vi "Read Image.vi"(0 "image in":refnum<class "MSC Image.lvclass">, 1 "image path":path, 5 "error in (no error)":errorcluster, 8 "read image properties":bool, 10 "image properties path":path) -> (14 "image out":refnum<class "MSC Image.lvclass">, 19 "error out":errorcluster)   [LabVIEW 2014, in "MSC Image.lvclass"]
doc: "Reads an image from the HD. If \"read image properties\" is set to TRUE, a previously created property file (.ini) is read and applied to the image.\n\nSupported formats:\nWindows bitmaps, JPEG, JPEG 2000, Portable Network Graphics, Portable image format, Sun rasters, TIFF"
uses:
  MSC Image.lvclass
  MSC Image.lvclass/MSC Image.ctl
  controls/INI Image Properties.vi
  controls/Size.ctl
  controls/Image Type.ctl
  <userlib>/_OpenG.lib/file/file.llb/Strip Path Extension - Path__ogtk.vi
  Dependencies/x86/MSC I Process32.dll
  <vilib>/Utility/config.llb/NI_LVConfig.lvlib
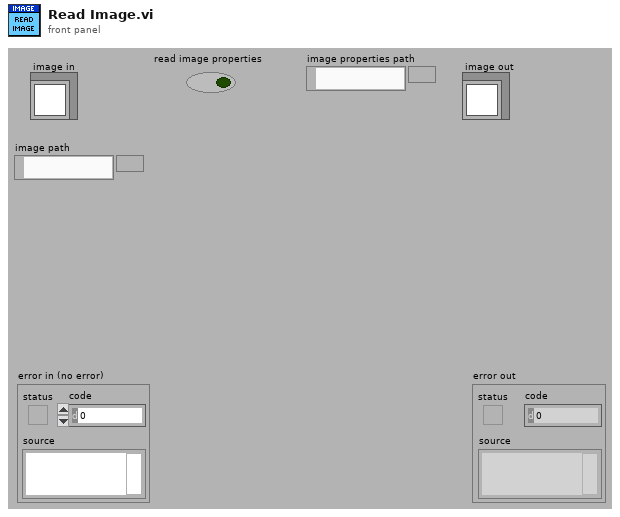
[diagram p1: front panel]
types:
  T1 = typedef "Image.ctl" = cluster{"Pointer":u64, "Size":T2, "Image Type":T3, "Time Stamp":timestamp, "Variant":variant}
  T2 = typedef "Size.ctl" = cluster{"Cols":i32, "Rows":i32}
  T3 = typedef "Image Type.ctl" = i32
  T4 = typedef "MSC Image.lvclass/INI Image Properties.vi" = cluster{"Size":T5, "Image Type":T6, "Timestamp":string, "Variant":variant}
  T5 = typedef "MSC Image.lvclass/Size.ctl" = cluster{"Cols":i32, "Rows":i32}
  T6 = typedef "MSC Image.lvclass/Image Type.ctl" = i32
  T7 = typedef "NI_LVConfig.lvlib/Config Data RefNum.ctl" = refnum<k1>
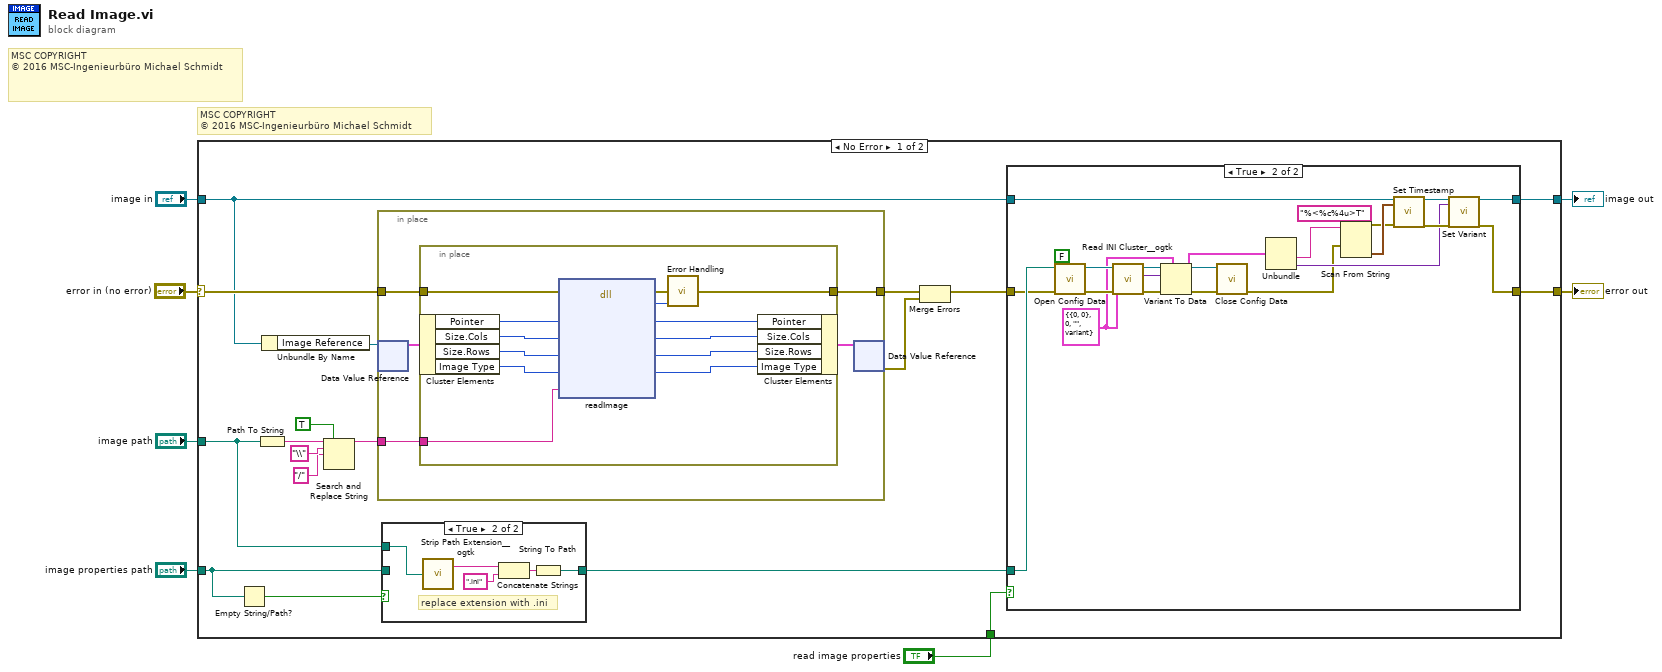
[diagram p0: block diagram]
diagram:
  # "MSC COPYRIGHT\n© 2016 MSC-Ingenieurbüro Michael Schmidt"
  # "MSC COPYRIGHT\n© 2016 MSC-Ingenieurbüro Michael Schmidt"
  # "MSC COPYRIGHT\n© 2016 MSC-Ingenieurbüro Michael Schmidt"
  n1 = case shown="No Error" "error in (no error)" {
    selector: "error in (no error)" -> [w22 w75]
    tunnel: [w13 w75] -> w6
    tunnel: [w15 w74] -> w4
    tunnel: "image in" -> [w16 w74]
    tunnel: "image path" -> [w9 _]
    tunnel: "image properties path" -> [w11 _]
    tunnel: "read image properties" -> [w8 _]
    frame No Error {
      n2 = Empty String/Path?(string/path=w11) -> (empty?=w12:bool)
      n3 = Path To String(path=w9) -> (string=w18:string)
      n4 = Unbundle By Name(w16) -> ("Image Reference"=w25:refnum<data-value>)
      n5 = Search and Replace String(replace all?=TRUE ("replace all? (F)"), input string=w18, search string="\\", replace string="/" ("replace string (\"\")")) -> (result string=w17:string)  [unwired: 4 in, 3 out]
      n6 = in-place {
        in-place-border: w22 -> [w58]
        in-place-border: [w57] -> w24
        in-place-border: w17 -> [w56]
        n7 = in-place-dvr #1(w25) -> (w59:T1)  [unwired: 1 out]
        n8 = in-place {
          in-place-border: w58 -> [w61]
          in-place-border: [w68] -> w57
          in-place-border: w56 -> [w62]
          n9 = in-place-cluster #2(w59) -> ("Pointer"=w71:u64, "Size.Cols"=w72:i32, "Size.Rows"=w73:i32, "Image Type"=w65:T3)
          n10 = dll-call lib="C:/Users/MSC/LabVIEW Projekte/LV 2014/MSC I-Process/user.lib/MSC-I Process/Dependencies/x86/MSC I Process*.dll" fn="readImage"(error in=w61, "pointer"=w71, "cols"=w72, "rows"=w73, "type"=w65, "pathString"=w62) -> (error out=w69:errorcluster, "error"=w70:i32, "pointer"=w63:u64, "cols"=w67:i32, "rows"=w66:i32, "type"=w64:i32)  [unwired: 3 in, 1 out]
          n11 = call "Error Handling.vi"("error in (no error)"=w69, "return type"=w70) -> ("error out"=w68:errorcluster)  [unwired: 12 in, 1 out]
          n12 = in-place-cluster #2("Pointer"=w63, "Size.Cols"=w67, "Size.Rows"=w66, "Image Type"=w64) -> (w60:T1)
        }
        n13 = in-place-dvr #1(w60) -> (w23:errorcluster)  [unwired: 1 out]
      }
      n14 = case shown="True" w12 {
        tunnel: w11 -> [w26 _]
        tunnel: [w26 w27] -> w10
        tunnel: w9 -> [_ w31]
        frame False {
        }
        frame True {
          # "replace extension with .ini"
          n15 = call-poly <userlib>:"Strip Path Extension__ogtk.vi"("path"=w31) -> ("root"=w30:string)  [unwired: 1 out]
          n16 = Concatenate Strings(w30, ".ini" ("string")) -> (w28:string)
          n17 = String To Path(string=w28) -> (path=w27:path)
        }
      }
      n18 = Merge Errors(w24, w23) -> (w14:errorcluster)
      n19 = case shown="True" w8 {
        tunnel: w16 -> [w33 w55]
        tunnel: [w33 w53] -> w15
        tunnel: w14 -> [w32 w44]
        tunnel: [w32 w52] -> w13
        tunnel: w10 -> [_ w45]
        frame False {
        }
        frame True {
          w42 = T4 {"Size"={"Cols"=0, "Rows"=0}, "Image Type"=0, "Timestamp"="", "Variant"=variant} ("CSV Image Properties")
          n20 = call <vilib>:"Open Config Data.vi"("error in (no error)"=w44, "create file if necessary (T)"=FALSE, "configuration file path"=w45) -> ("error out"=w47:errorcluster, "refnum"=w46:T7)  [unwired: 6 in, 1 out]
          n21 = call <userlib>:"Read INI Cluster__ogtk.vi"("error in (no error)"=w47, "INI Fomatted Cluster Type"=w42, "refnum"=w46) -> ("error out"=w40:errorcluster, "INI Fomatted Cluster"=w41:variant, "dup refnum"=w48:T7)  [unwired: 4 in, 2 out]
          n22 = Variant To Data(error in=w40, type=w42, Variant=w41) -> (data=w38:T4, error out=w39:errorcluster)
          n23 = call <vilib>:"Close Config Data.vi"("error in (no error)"=w39, "refnum"=w48) -> ("error out"=w35:errorcluster)  [unwired: 8 in, 1 out]
          n24 = Unbundle(w38) -> ("Timestamp"=w37:string, "Variant"=w36:variant)  [unwired: 2 out]
          n25 = Scan From String(format string="%<%c%4u>T", input string=w37, error in=w35) -> (error out=w34:errorcluster, output 1=w49:timestamp)  [unwired: 2 in, 2 out]
          n26 = call-dynamic "Set Timestamp.vi"("image in"=w55, "Time Stamp"=w49, "error in (no error)"=w34) -> ("image out"=w54:refnum<class "MSC Image.lvclass">, "error out"=w51:errorcluster)  [unwired: 15 in]
          n27 = call-dynamic "Set Variant.vi"("image in"=w54, "Variant"=w36, "error in (no error)"=w51) -> ("image out"=w53:refnum<class "MSC Image.lvclass">, "error out"=w52:errorcluster)  [unwired: 15 in]
        }
      }
    }
    frame Error {
    }
  }
  "error out" <- w6
  "image out" <- w4
